vi "LJM_ReadRaw.vi"(8 "error in":errorcluster, 10 "NumBytes":i32, 11 "Handle In":i32) -> (0 "error out":errorcluster, 1 "Data":u8[](array[numeric]), 3 "Handle Out":i32)   [LabVIEW 2020]
uses:
  LabJackM.framework
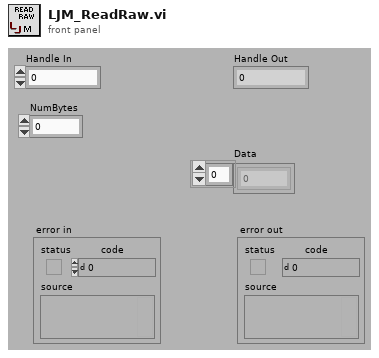
[diagram p1: front panel]
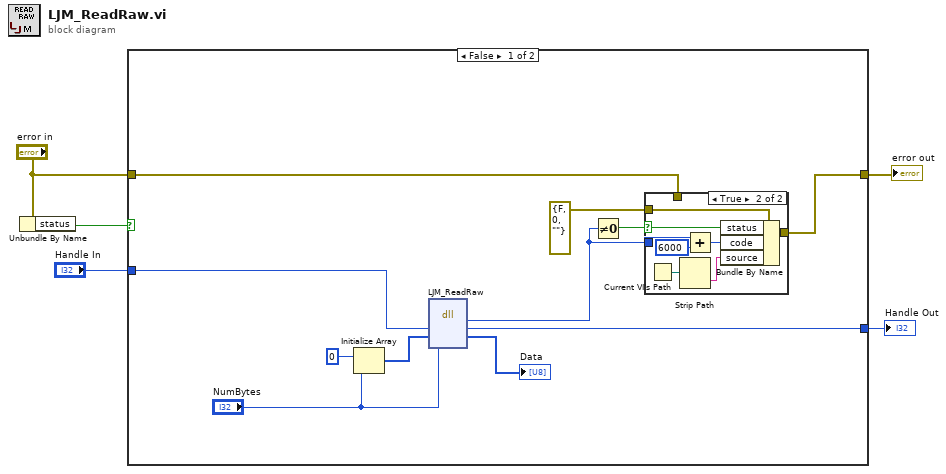
[diagram p0: block diagram]
diagram:
  n1 = Unbundle By Name("error in") -> ("status"=w5:bool)
  n2 = case shown="False" w5 {
    tunnel: "error in" -> [w12 w27]
    tunnel: [w13 w27] -> w3
    tunnel: [w11 w26] -> w2
    tunnel: "Handle In" -> [w10 w26]
    frame False {
      n3 = Initialize Array(u8 0 ("Element Data"), "NumBytes") -> (w7:u8[])
      n4 = dll-call lib="LabJackM.framework" fn="LJM_ReadRaw"("Handle"=w10, "Data"=w7, "NumBytes"="NumBytes") -> ("return type"=w16:i32, "Handle"=w11:i32, "Data"=→"Data":u8[])  [unwired: 4 in, 2 out]
      n5 = Not Equal To 0?(x=w16) -> (x != 0?=w15:bool)
      n6 = case shown="True" w15 {
        selector: w15 -> [_ w24]
        tunnel: [w17 w25] -> w13
        tunnel: errorcluster {"status"=FALSE, "code"=0, "source"=""} ("error IO") -> [_ w23]
        tunnel: w16 -> [_ w19]
        tunnel: w12 -> [w17 _]
        frame False {
        }
        frame True {
          n7 = Current VI's Path() -> (path=w21:path)
          n8 = Strip Path(path=w21) -> (name=w22:string)  [unwired: 1 out]
          n9 = Add(x=w19, y=6000) -> (x+y=w20:i32)
          n10 = Bundle By Name(cluster=w23, "status"=w24, "code"=w20, "source"=w22) -> (w25:errorcluster)
        }
      }
    }
    frame True {
    }
  }
  "error out" <- w3
  "Handle Out" <- w2
